vi "PrintDialog.vi"() -> ()   [LabVIEW 2013]
doc: "This VI calls a CIN that displays the Windows Print Setup dialog."
panel:
  out "Success ?":bool
  # "This VI displays the Windows Print Setup dialog."
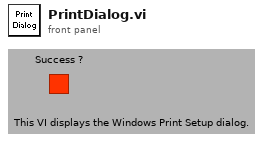
[diagram p1: front panel]
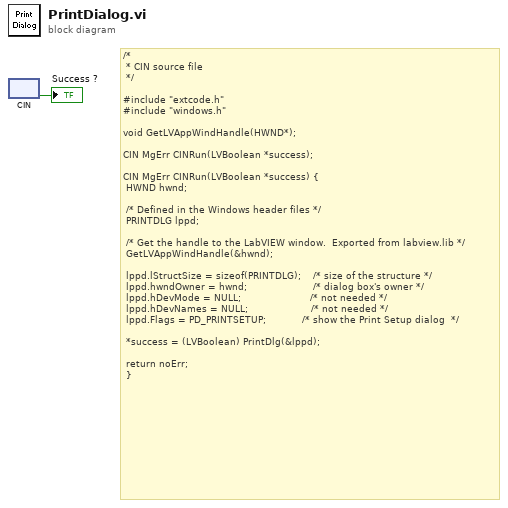
[diagram p0: block diagram]
diagram:
  # "/*\n * CIN source file \n */\n\n#include \"extcode.h\"\n#include \"windows.h\"\n\nvoid GetLVAppWindHandle(HWND*);\n\nCIN MgErr CINRun(LVBoolean *success);\n\nCIN MgErr CINRun(LVBoolean *success) {\n\tHWND hwnd;\n\t\n\t/* Defined in the Windows header files */\n\tPRINTDLG lppd; \n\t\n\t/* Get the handle to the LabVIEW window.  Exported from labview.lib */\n\tGetLVAppWindHandle(&hwnd);\n\n\tlppd.lStructSize = sizeof(PRINTDLG);\t   /* size of the structure */\n\tlppd.hwndOwner = hwnd;\t\t\t\t\t                 /* dialog box's owner */\n\tlppd.hDevMode = NULL;\t\t\t\t\t                  /* not needed */\n\tlppd.hDevNames = NULL;\t\t\t\t\t                /* not needed */\n\tlppd.Flags = PD_PRINTSETUP;\t\t\t\t        /* show the Print Setup dialog  */\n\t\n\t*success = (LVBoolean) PrintDlg(&lppd);\t\t\n\n\treturn noErr;\n\t}"
  n1 = cin() -> (→"Success ?":bool)  [unwired: 1 in]
